vi "PID power calc.vi"(7 "DAQq cluster in":T1 {"temp"."utility"."therm volt" format="%_6g"; "temp"."utility"."heat volt in" format="%_6g"; "temp"."utility"."heat volt out" format="%_6g"; "temp"."utility"."power out" format="%_6g"; "temp"."utility"."H Vmax" format="%_6g"; "temp"."T exec"."man power" format="%_6g"; "temp"."T exec"."exec setpoint" format="%_6g"; "temp"."T params"."Settle Time" step=1.0; "temp"."T params"."Settle Bandwidth" step=0.01; "temp"."T params"."Derivative Tme" step=0.01; "temp"."T params"."Integral Time" step=1.0; "temp"."T params"."Control Bandwidth" step=0.1; "temp"."T params"."Setpoint" step=0.1; "temp"."T status"."Setpoint" format="%_6g"; "temp"."T status"."Power" format="%_6g"; "temp"."T status"."Temp" format="%_6g"}) -> (8 "DAQ cluster out":T1 {"temp"."utility"."therm volt" format="%_6g"; "temp"."utility"."heat volt in" format="%_6g"; "temp"."utility"."heat volt out" format="%_6g"; "temp"."utility"."power out" format="%_6g"; "temp"."utility"."H Vmax" format="%_6g"; "temp"."T exec"."man power" format="%_6g"; "temp"."T exec"."exec setpoint" format="%_6g"; "temp"."T params"."Settle Time" step=1.0; "temp"."T params"."Settle Bandwidth" step=0.01; "temp"."T params"."Derivative Tme" step=0.01; "temp"."T params"."Integral Time" step=1.0; "temp"."T params"."Control Bandwidth" step=0.1; "temp"."T params"."Setpoint" step=0.1; "temp"."T status"."Setpoint" format="%_6g"; "temp"."T status"."Power" format="%_6g"; "temp"."T status"."Temp" format="%_6g"})   [LabVIEW 2019]
doc: "This is a Bug C(T) subVI.\n\nThis subVI is one of the states of the DAQ state machine in the bug experiment.\n\nThis state does a PID calulation to determine the power to output.\n\nIt proceeds to output power next.\n\nPaul K Dixon\nP3600\nCSUSB Physics"
uses:
  typedefs/DAQ state cluster.ctl
  typedefs/DAQ state enum.ctl
  typedefs/temp cont cluster.ctl
  typedefs/temp exec cluster.ctl
  typedefs/temp mode enum.ctl
  typedefs/temp indicator.ctl
  typedefs/temp control status.ctl
  typedefs/PID control parameters.ctl
  typedefs/temp cont utility.ctl
  typedefs/measurement.ctl
  typedefs/wvfm acq params.ctl
panel:
  out "in settle band":bool
  out "in control band":bool
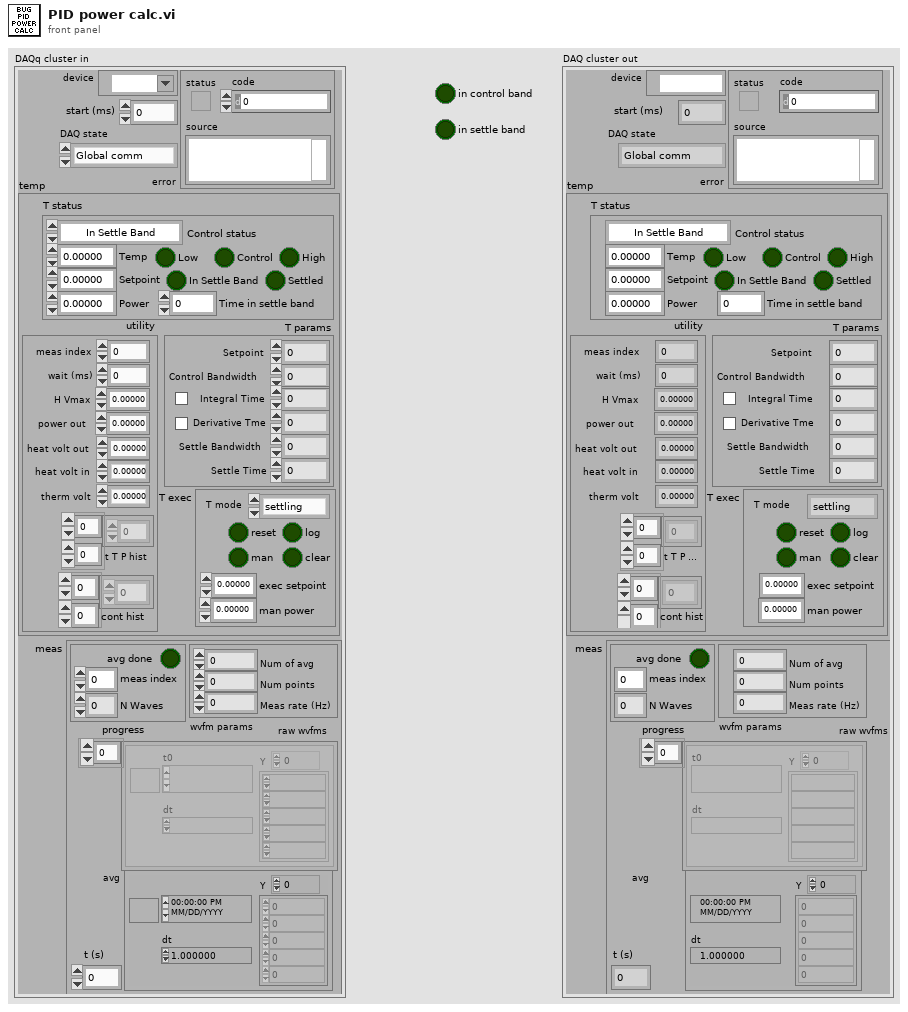
[diagram p1: front panel]
types:
  T1 = typedef "DAQ state cluster.ctl" = cluster{"DAQ state":T2, "temp":T3, "meas":T10, "device":tag, "error":errorcluster, "start (ms)":i32}
  T2 = typedef "DAQ state enum.ctl" = enum16{"Global comm", "Meas T & P", "PID power calc", "Man Power set", "Output Power", "Wait", "Meas wvfm", "Avg wvfm", "Exit"}
  T3 = typedef "temp cont cluster.ctl" = cluster{"T exec":T4, "T status":T6, "T params":T8, "utility":T9}
  T4 = typedef "temp exec cluster.ctl" = cluster{"T mode":T5, "exec setpoint":dbl, "reset":bool, "man power":dbl, "man":bool, "log":bool, "clear":bool}
  T5 = typedef "temp mode enum.ctl" = enum16{"settling", "measuring", "holding", "Exit"}
  T6 = typedef "temp indicator.ctl" = cluster{"Control status":T7, "Temp":dbl, "Power":dbl, "Time in settle band":dbl, "Settled":bool, "Low":bool, "High":bool, "Setpoint":dbl, "Control":bool, "In Settle Band":bool}
  T7 = typedef "temp control status.ctl" = enum16{"In Settle Band", "In Control Band", "Below Control Band", "Above Control Band"}
  T8 = typedef "PID control parameters.ctl" = cluster{"Setpoint":dbl, "Control Bandwidth":dbl, "Integral Time":dbl, "Int\nON":bool, "Derivative Tme":dbl, "Der\nON":bool, "Settle Bandwidth":dbl, "Settle Time":dbl}
  T9 = typedef "temp cont utility.ctl" = cluster{"meas index":i32, "wait (ms)":i32, "H Vmax":dbl, "power out":dbl, "heat volt out":dbl, "heat volt in":dbl, "therm volt":dbl, "t T P hist":dbl[][], "cont hist":dbl[][]}
  T10 = typedef "measurement.ctl" = cluster{"wvfm params":T11, "avg":waveform(dbl), "raw wvfms":waveform(dbl)[], "progress":cluster{"avg done":bool, "meas index":i32, "N waves":i32}, "t (s)":dbl}
  T11 = typedef "wvfm acq params.ctl" = cluster{"Num of avg":i32, "Num points":i32, "Meas rate (Hz)":dbl}
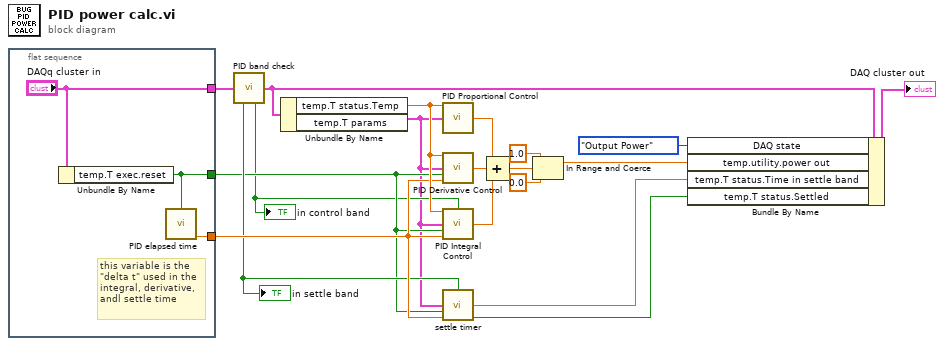
[diagram p0: block diagram]
diagram:
  n1 = flat-sequence {
    tunnel: [w22] -> w9
    tunnel: [w21] -> w7
    tunnel: ["DAQq cluster in"] -> w2
    frame #0 {
      # "this variable is the \n\"delta t\" used in the\nintegral, derivative,\nandl settle time"
      n2 = Unbundle By Name("DAQq cluster in") -> ("temp.T exec.reset"=w21:bool)
      n3 = call "PID elapsed time.vi"("reset"=w21) -> ("elaspsed time (sec)"=w22:dbl)  [unwired: 13 in, 1 out]
    }
  }
  n4 = call "PID band check.vi"("DAQ cluster in"=w2) -> ("DAQ cluster out"=w18:T1, "In SB"=w8:bool, "In CB"=w6:bool)  [unwired: 12 in]
  "in control band" <- w6
  "in settle band" <- w8
  n5 = Unbundle By Name(w18) -> ("temp.T status.Temp"=w10:dbl, "temp.T params"=w3:T8)
  n6 = call "PID Proportional Control.vi"("Temp"=w10, "Control Parameters"=w3) -> ("Proportional Power"=w16:dbl)  [unwired: 13 in]
  n7 = call "PID Derivative Control.vi"("Temp In (deg C)"=w10, "Control Parameters"=w3, "reset"=w7, "delta t"=w9) -> ("Derivative Power"=w17:dbl)  [unwired: 11 in]
  n8 = call "PID Integral Control.vi"("Temp In (deg C)"=w10, "in control band"=w6, "Control Parameters"=w3, "reset"=w7, "delta t"=w9) -> ("Integral Power"=w15:dbl)  [unwired: 10 in]
  n9 = call "settle timer.vi"("in settle band"=w8, "Control Parameters"=w3, "reset"=w7, "delta t"=w9) -> ("time in settle band"=w5:dbl, "settled"=w4:bool)  [unwired: 10 in]
  n10 = Compound Arithmetic op=ADD(w16, w17, w15) -> (w14:dbl)
  n11 = In Range and Coerce(upper limit=1.0, x=w14, lower limit=0.0) -> (coerced(x)=w11:dbl)  [unwired: 1 out]
  n12 = Bundle By Name(cluster=w18, "DAQ state"=DAQ_state_enum."Output Power", "temp.utility.power out"=w11, "temp.T status.Time in settle band"=w5, "temp.T status.Settled"=w4) -> (→"DAQ cluster out":T1)
